vi "Stop Task.vi"(8 "error in":errorcluster, 10 "Task Ident":string, 11 "Series Actor in":refnum<class "Series Actor.lvclass">) -> (0 "error out":errorcluster, 3 "Series Actor out":refnum<class "Series Actor.lvclass">)   [LabVIEW 2023, in "Series Actor.lvlib" / "Series Actor.lvclass"]
uses:
  Series Actor.lvclass
  Series Actor.lvclass/Series Actor.ctl
  <vilib>/ActorFramework/Message Enqueuer/Message Enqueuer.lvclass/Message Enqueuer.ctl
  <vilib>/ActorFramework/Message Enqueuer/Enqueue.vi
  Task/ITask Actor/ITask Actor Messages/Stop Do Msg/Stop Do Msg.lvclass
  <vilib>/Utility/error.llb/Error Cluster From Error Code.vi
  <vilib>/Utility/LVClass/Get LV Class Name.vi
  <resource>/AFDebug/Generate Trace for Message.vi
  <vilib>/ActorFramework/Message Priority Queue/Priority Enqueue.vi
  <vilib>/ErrorRing/Error Ring.xnode
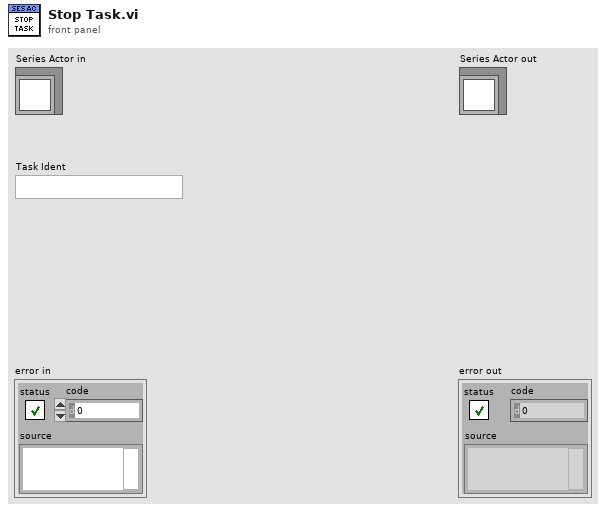
[diagram p1: front panel]
types:
  T1 = map{string, refnum<class "Message Enqueuer.lvclass">}
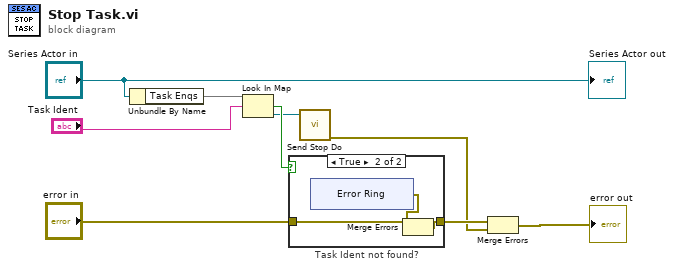
[diagram p0: block diagram]
diagram:
  n1 = Unbundle By Name("Series Actor in") -> ("Task Enqs"=w5:T1)
  n2 = Look In Map(map=w5, key="Task Ident") -> (key not found?=w4:bool, value=w3:refnum<class "Message Enqueuer.lvclass">)  [unwired: 1 in]
  n3 = case "Task Ident not found?" shown="True" w4 {
    tunnel: "error in" -> [w10 w13]
    tunnel: [w10 w11] -> w2
    frame False {
    }
    frame True {
      n4 = xnode "Error Ring"() -> ("error out"=w12:errorcluster)
      n5 = Merge Errors(w13, w12) -> (w11:errorcluster)
    }
  }
  n6 = call "Send Stop Do.vi"("Message Enqueuer"=w3) -> ("error out"=w1:errorcluster)  [unwired: 9 in, 1 out]
  n7 = Merge Errors(w2, w1) -> (→"error out":errorcluster)
  "Series Actor out" <- "Series Actor in"
